vi "Example_Lockin.vi"() -> ()   [LabVIEW 2016]
uses:
  Instrument.Lockin/Instrument.Lockin.lvclass
  <userlib>/LevyLab/LV to ITX/LVtoITX.lvclass
  LockinDAQ/Typedefs/AO_Amp-array.ctl
  LockinDAQ/LockinDAQ.lvclass
  LockinDAQ/Typedefs/AO_DC-array.ctl
  LockinDAQ/Typedefs/AO_phi-array.ctl
  LockinDAQ/Typedefs/Function-array.ctl
  LockinDAQ/Typedefs/AO_f-array.ctl
  LockinDAQ/Typedefs/AO-cluster.ctl
  LockinDAQ/Typedefs/REF_f-array.ctl
  LockinDAQ/Typedefs/REF_phi-array.ctl
  LockinDAQ/Typedefs/REF-cluster.ctl
  LockinDAQ/Typedefs/Function-enum.ctl
panel:
  in  "Channels: Lockin":T1 {"REF phi (°)" format="%#_3g"}
  out "Lockin vs time":cluster{timestamp[], dbl[]}(graph)
  out "Lockin vs parameter":cluster{"Y":dbl[], "Y":dbl[]}(graph)
  in  "step":dbl=0.025
  in  "end":dbl=0.1
  in  "start":dbl
  in  "Channels: AO":T4 {"AO f (Hz)" min=0.001 max=10000.0; "AO DC (V)" format="%.3p"; "AO Amp (V)" format="%.3p"}
  # "Lockin Example: Lockin\nMake Sure Lockin Program is running!"
  # "1"
  # "2"
  # "3"
  # "4"
  # "5"
  # "6"
  # "7"
  # "8"
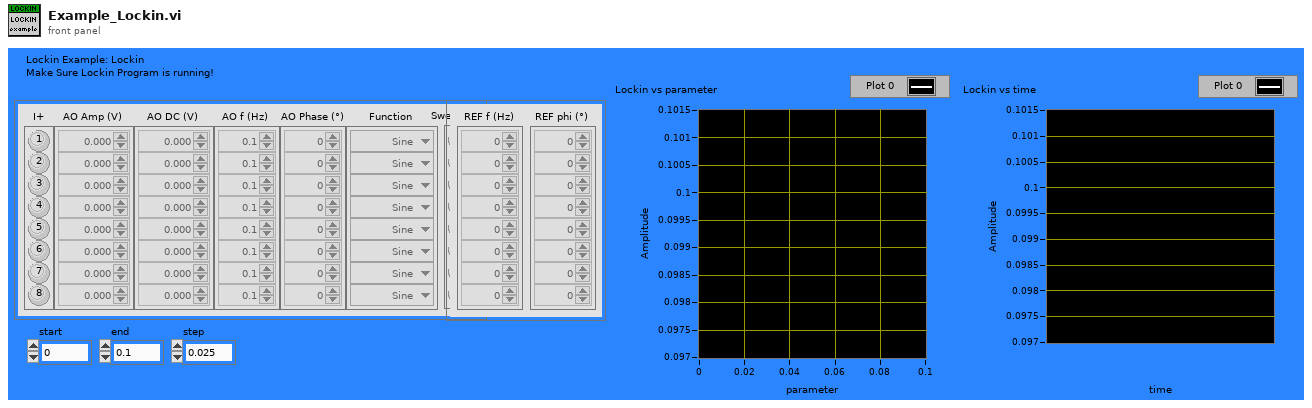
[diagram p1: front panel]
types:
  T1 = typedef "LockinDAQ.lvclass/REF-cluster.ctl" = cluster{"REF f (Hz)":T2, "REF phi (°)":T3}
  T2 = typedef "LockinDAQ.lvclass/REF_f-array.ctl" = dbl[]
  T3 = typedef "LockinDAQ.lvclass/REF_phi-array.ctl" = dbl[]
  T4 = typedef "LockinDAQ.lvclass/AO-cluster.ctl" = cluster{"AO Amp (V)":T5, "AO DC (V)":T6, "AO f (Hz)":T7, "AO Phase (°)":T8, "Function":T9, "I+":bool[], "Sweeping":bool[]}
  T5 = typedef "LockinDAQ.lvclass/AO_Amp-array.ctl" = dbl[]
  T6 = typedef "LockinDAQ.lvclass/AO_DC-array.ctl" = dbl[]
  T7 = typedef "LockinDAQ.lvclass/AO_f-array.ctl" = dbl[]
  T8 = typedef "LockinDAQ.lvclass/AO_phi-array.ctl" = dbl[]
  T9 = typedef "LockinDAQ.lvclass/Function-array.ctl" = T10[]
  T10 = typedef "LockinDAQ.lvclass/Function-enum.ctl" = enum16{"Sine", "Triangle", "Square", "Sawtooth"}
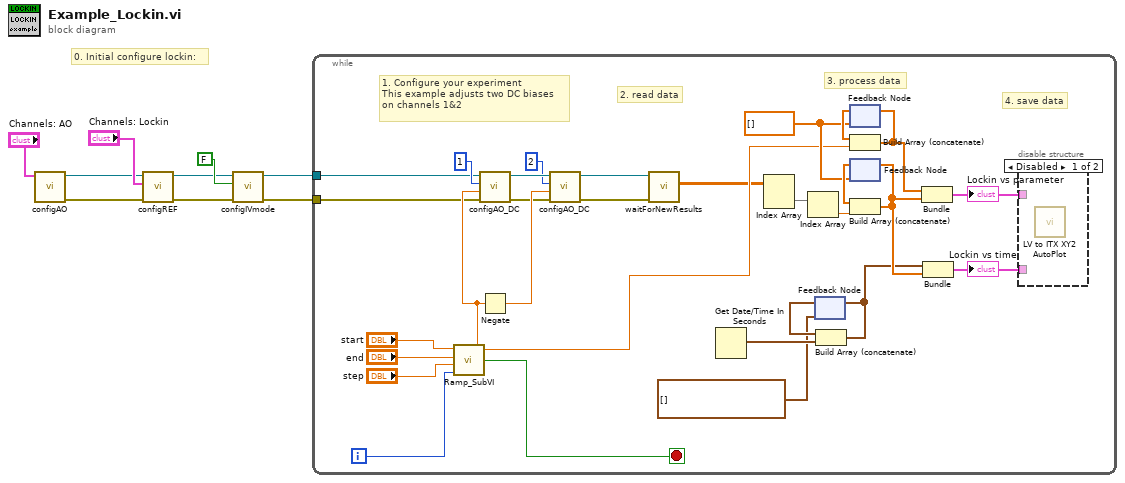
[diagram p0: block diagram]
diagram:
  # "0. Initial configure lockin:"
  n1 = call "configAO.vi"("Channels: AO"="Channels: AO") -> ("error out"=w6:errorcluster, "Instrument.Lockin out"=w7:refnum<class "Instrument.Lockin.lvclass">)  [unwired: 9 in]
  n2 = call "configREF.vi"("error in (no error)"=w6, "Channels: Lockin in"="Channels: Lockin", "Instrument.Lockin in"=w7) -> ("error out"=w1:errorcluster, "Instrument.Lockin out"=w4:refnum<class "Instrument.Lockin.lvclass">)  [unwired: 7 in]
  n3 = call "configIVmode.vi"("error in (no error)"=w1, "IV mode"=FALSE, "Instrument.Lockin in"=w4) -> ("error out"=w2:errorcluster, "Instrument.Lockin out"=w3:refnum<class "Instrument.Lockin.lvclass">)  [unwired: 7 in]
  n4 = while {
    tunnel: w2 -> [w14]
    tunnel: w3 -> [w13]
    i -> [w35]
    stop <- w38 stop-if-true
    w22 = dbl[] []
    # "4. save data"
    # "3. process data"
    # "2. read data"
    # "1. Configure your experiment\nThis example adjusts two DC biases\non channels 1&2"
    n5 = call <userlib>:"Ramp_SubVI.vi"("index"=w35, "step"="step", "end"="end", "start"="start") -> ("Stop?"=w38:bool, "Numeric"=w17:dbl)  [unwired: 1 in]
    n6 = call "configAO_DC.vi"("error in (no error)"=w14, "DC (V)"=w17, "AO Channel"=1, "Instrument.Lockin in"=w13) -> ("error out"=w15:errorcluster, "Instrument.Lockin out"=w20:refnum<class "Instrument.Lockin.lvclass">)  [unwired: 6 in]
    n7 = Negate(x=w17) -> (-x=w16:dbl)
    n8 = call "configAO_DC.vi"("error in (no error)"=w15, "DC (V)"=w16, "AO Channel"=2, "Instrument.Lockin in"=w20) -> ("error out"=w11:errorcluster, "Instrument.Lockin out"=w10:refnum<class "Instrument.Lockin.lvclass">)  [unwired: 6 in]
    n9 = call "waitForNewResults.vi"("error in (no error)"=w11, "Instrument.Lockin in"=w10) -> ("Results"=w12:dbl[][])  [unwired: 7 in, 2 out]
    n10 = Get Date/Time In Seconds() -> (seconds since 1Jan1904=w25:timestamp)
    n11 = Index Array(array=w12) -> (element=w31:dbl[])  [unwired: 2 in]
    n12 = Index Array(array=w31) -> (element=w30:dbl)  [unwired: 1 in]
    n13 = feedback #1(timestamp[] []) -> (w23:timestamp[])
    n14 = Build Array (concatenate)(w23, w25) -> (w24:timestamp[])
    n15 = feedback-in #1(w24) -> ()
    n16 = feedback #2(w22) -> (w27:dbl[])
    n17 = Build Array (concatenate)(w27, w17) -> (w26:dbl[])
    n18 = feedback-in #2(w26) -> ()
    n19 = feedback #3(w22) -> (w29:dbl[])
    n20 = Build Array (concatenate)(w29, w30) -> (w28:dbl[])
    n21 = feedback-in #3(w28) -> ()
    n22 = Bundle(w26, w28) -> (w33:cluster{dbl[], dbl[]})  [unwired: 1 in]
    "Lockin vs parameter" <- w33
    n23 = Bundle(w24, w28) -> (w32:cluster{timestamp[], dbl[]})  [unwired: 1 in]
    "Lockin vs time" <- w32
    n24 = disable-structure shown="Disabled" {
      disable-tunnel: w33 -> [_ _]
      disable-tunnel: w32 -> [_ _]
      frame Disabled {
        n25 = call <userlib>:"LV to ITX XY2 AutoPlot.vi"() -> ()  [unwired: 15 in, 1 out]
      }
      frame Enabled {
      }
    }
  }
